vi "dfd_Structure Group Four Five Internal Conversion.vi"(8 "error in (no error)":errorcluster, 10 "target structure":T2, 11 "filter coef in":T1) -> (0 "error out":errorcluster, 3 "filter coef out":T1)   [LabVIEW 2017, in "NI_DigFilterLicensed.lvlib"]
uses:
  <vilib>/addons/Digital Filter Design/NI_DigFilterLicensed.lvlib
  <vilib>/addons/Digital Filter Design/_Objects.llb/DFD Filter Coef.ctl
  <vilib>/addons/Digital Filter Design/_Objects.llb/DFD Filter Structure Type Selector.ctl
  <vilib>/addons/Digital Filter Design/_Objects.llb/DFD Lattice Type.ctl
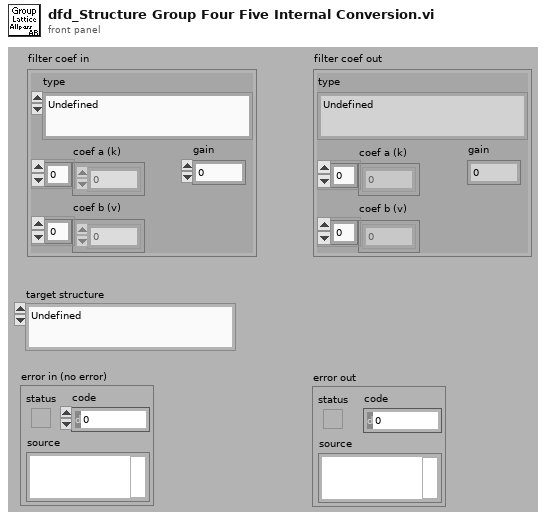
[diagram p1: front panel]
types:
  T1 = typedef "NI_DigFilterLicensed.lvlib/DFD Filter Coef.ctl" = cluster{"type":T2, "gain":dbl, "coef a (k)":dbl[], "coef b (v)":dbl[]}
  T2 = typedef "NI_DigFilterLicensed.lvlib/DFD Filter Structure Type Selector.ctl" = enum16{"Undefined", "FIR Direct Form", "FIR Direct Form Transposed", "FIR Symmetric", "FIR Antisymmetric", "IIR Direct Form I", "IIR Direct Form I Transposed", "IIR Direct Form II", "IIR Direct Form II Transposed", "IIR Cascaded Second Order Sections Form I", "IIR Cascaded Second Order Sections Form I Transposed", "IIR Cascaded Second Order Sections Form II", "IIR Cascaded Second Order Sections Form II Transposed", "Lattice Allpass (basic sections)", "Lattice Allpass (one multiplier sections)", "Lattice Allpass (normalized sections)", "Lattice AR (basic sections)", "Lattice AR (one multiplier sections)", "Lattice AR (normalized sections)", "Lattice MA (minimum phase)", "Lattice MA (maximum phase)", "Lattice ARMA (basic sections)", "Lattice ARMA (one multiplier sections)", "Lattice ARMA (normalized sections)"}
  T3 = typedef "NI_DigFilterLicensed.lvlib/DFD Lattice Type.ctl" = enum16{"Undefined", "Lattice Allpass", "Lattice AR", "Lattice MA (min)", "Lattice MA (max)", "Lattice ARMA"}
  T4 = enum16{"Undefined", "Basic", "One Multiplier", "Normalized"}
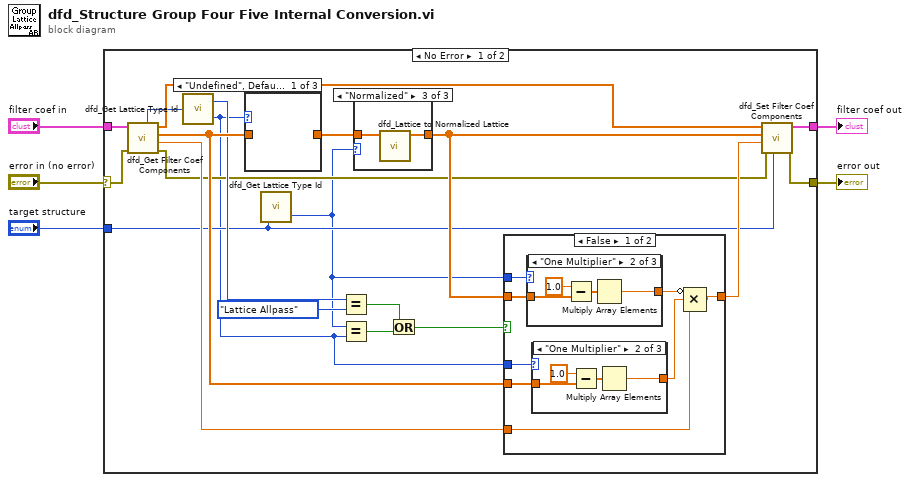
[diagram p0: block diagram]
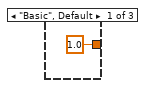
[diagram p2: hidden frame]
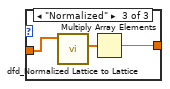
[diagram p3: hidden frame]
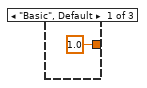
[diagram p4: hidden frame]
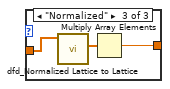
[diagram p5: hidden frame]
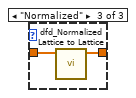
[diagram p10: hidden frame]
diagram:
  n1 = case shown="No Error" "error in (no error)" {
    selector: "error in (no error)" -> [w21 w57]
    tunnel: [w19 w57] -> w1
    tunnel: [w20 w58] -> w2
    tunnel: "filter coef in" -> [w23 w58]
    tunnel: "target structure" -> [w8 _]
    frame No Error {
      n2 = call <vilib>:"dfd_Get Filter Coef Components.vi"("error in (no error)"=w21, "filter coef"=w23) -> ("error out"=w9:errorcluster, "gain"=w17:dbl, "coef a (k)"=w15:dbl[], "coef b (v)"=w25:dbl[], "type"=w22:T2)  [unwired: 5 out]
      n3 = call <vilib>:"dfd_Get Lattice Type Id.vi"("structure type"=w22) -> ("lattice type"=w14:T3, "section type"=w6:T4)
      n4 = case shown="\"Undefined\", Default" w6 {
        tunnel: w15 -> [_ w54 w56]
        tunnel: [_ w54 w55] -> w24
        frame "Undefined", Default {
        }
        frame "Basic", "One Multiplier" {
        }
        frame "Normalized" {
          n5 = call <vilib>:"dfd_Normalized Lattice to Lattice.vi"("k & ^k"=w56) -> ("k [M~1]"=w55:dbl[])  [unwired: 10 out]
        }
      }
      n6 = call <vilib>:"dfd_Get Lattice Type Id.vi"("structure type"=w8) -> ("section type"=w7:T4)  [unwired: 1 out]
      n7 = Equal?(x=w14, y=DFD_Lattice_Type."Lattice Allpass") -> (x = y?=w10:bool)
      n8 = Equal?(x=w7, y=w6) -> (x = y?=w11:bool)
      n9 = case shown="\"Normalized\"" w7 {
        tunnel: w24 -> [_ w51 w53]
        tunnel: [_ w51 w52] -> w18
        frame "Undefined", Default {
        }
        frame "Basic", "One Multiplier" {
        }
        frame "Normalized" {
          n10 = call <vilib>:"dfd_Lattice to Normalized Lattice.vi"("k [M~1]"=w53) -> ("k & ^k"=w52:dbl[])  [unwired: 10 out]
        }
      }
      n11 = Or(x=w10, y=w11) -> (x .or. y?=w12:bool)
      n12 = case shown="False" w12 {
        tunnel: w7 -> [w33 _]
        tunnel: w18 -> [w32 _]
        tunnel: w17 -> [w26 w50]
        tunnel: [w30 w50] -> w16
        tunnel: w15 -> [w29 _]
        tunnel: w6 -> [w28 _]
        frame False {
          n13 = case shown="\"One Multiplier\"" w33 {
            tunnel: w32 -> [_ w44 w48]
            tunnel: [1.0 w43 w47] -> w31
            frame "Basic", Default {
            }
            frame "One Multiplier" {
              n14 = Subtract(x=1.0, y=w44) -> (x-y=w45:dbl[])
              n15 = Multiply Array Elements(1:w45) -> (0:w43:dbl)
            }
            frame "Normalized" {
              n16 = call <vilib>:"dfd_Normalized Lattice to Lattice.vi"("k & ^k"=w48) -> ("^k [M~1]"=w49:dbl[])  [unwired: 10 out]
              n17 = Multiply Array Elements(1:w49) -> (0:w47:dbl)
            }
          }
          n18 = case shown="\"One Multiplier\"" w28 {
            tunnel: w29 -> [_ w36 w40]
            tunnel: [1.0 w35 w39] -> w27
            frame "Basic", Default {
            }
            frame "One Multiplier" {
              n19 = Subtract(x=1.0, y=w36) -> (x-y=w37:dbl[])
              n20 = Multiply Array Elements(1:w37) -> (0:w35:dbl)
            }
            frame "Normalized" {
              n21 = call <vilib>:"dfd_Normalized Lattice to Lattice.vi"("k & ^k"=w40) -> ("^k [M~1]"=w41:dbl[])  [unwired: 10 out]
              n22 = Multiply Array Elements(1:w41) -> (0:w39:dbl)
            }
          }
          n23 = Compound Arithmetic op=MULTIPLY(invert w31, w27, w26) -> (w30:dbl)
        }
        frame True {
        }
      }
      n24 = call <vilib>:"dfd_Set Filter Coef Components.vi"("type"=w8, "error in (no error)"=w9, "gain"=w16, "coef a (k)"=w18, "coef b (v)"=w25) -> ("error out"=w19:errorcluster, "filter coef"=w20:T1)  [unwired: 5 out]
    }
    frame Error {
    }
  }
  "error out" <- w1
  "filter coef out" <- w2
